vi "subAddControl.vi"(0 "Input Symbol Stream":cdb[][](array[numeric]), 9 "Training Sequence":cdb[](array[numeric])=[0.7071067811865475+0.7071067811865475i, 0.7071067811865475+0.7071067811865475i, 0.7071067811865475+0.7071067811865475i, -0.7071067811865475-0.7071067811865475i, -0.7071067811865475-0.7071067811865475i, -0.7071067811865475-0.7071067811865475i, 0.7071067811865475+0.7071067811865475i, -0.7071067811865475-0.7071067811865475i, -0.7071067811865475-0.7071067811865475i, 0.7071067811865475+0.7071067811865475i, -0.7071067811865475-0.7071067811865475i, 0.7071067811865475+0.7071067811865475i, 0.7071067811865475+0.7071067811865475i, 0.7071067811865475+0.7071067811865475i, -0.7071067811865475-0.7071067811865475i, -0.7071067811865475-0.7071067811865475i, -0.7071067811865475-0.7071067811865475i, 0.7071067811865475+0.7071067811865475i, -0.7071067811865475-0.7071067811865475i, -0.7071067811865475-0.7071067811865475i, 0.7071067811865475+0.7071067811865475i, -0.7071067811865475-0.7071067811865475i, 0.7071067811865475+0.7071067811865475i, 0.7071067811865475+0.7071067811865475i, 0.7071067811865475+0.7071067811865475i, -0.7071067811865475-0.7071067811865475i, -0.7071067811865475-0.7071067811865475i, -0.7071067811865475-0.7071067811865475i, 0.7071067811865475+0.7071067811865475i, -0.7071067811865475-0.7071067811865475i, -0.7071067811865475-0.7071067811865475i, 0.7071067811865475+0.7071067811865475i, -0.7071067811865475-0.7071067811865475i, 0.7071067811865475+0.7071067811865475i, 0.7071067811865475+0.7071067811865475i, 0.7071067811865475+0.7071067811865475i, -0.7071067811865475-0.7071067811865475i, -0.7071067811865475-0.7071067811865475i, -0.7071067811865475-0.7071067811865475i, 0.7071067811865475+0.7071067811865475i, -0.7071067811865475-0.7071067811865475i, -0.7071067811865475-0.7071067811865475i, 0.7071067811865475+0.7071067811865475i, -0.7071067811865475-0.7071067811865475i] format="%#_3p", 11 "error in (no error)":errorcluster) -> (4 "Output Transmit \nPackets":cdb[][](array[numeric]), 15 "error out":errorcluster)   [LabVIEW 2011]
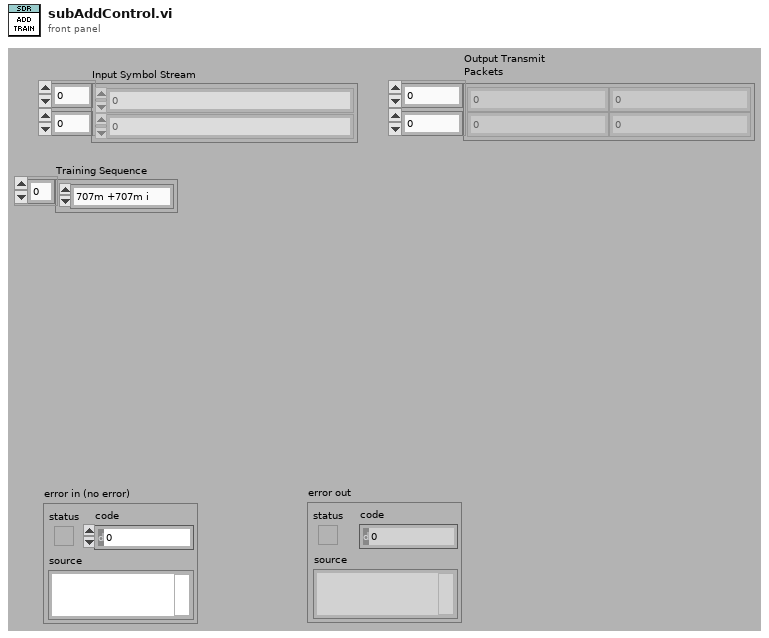
[diagram p1: front panel]
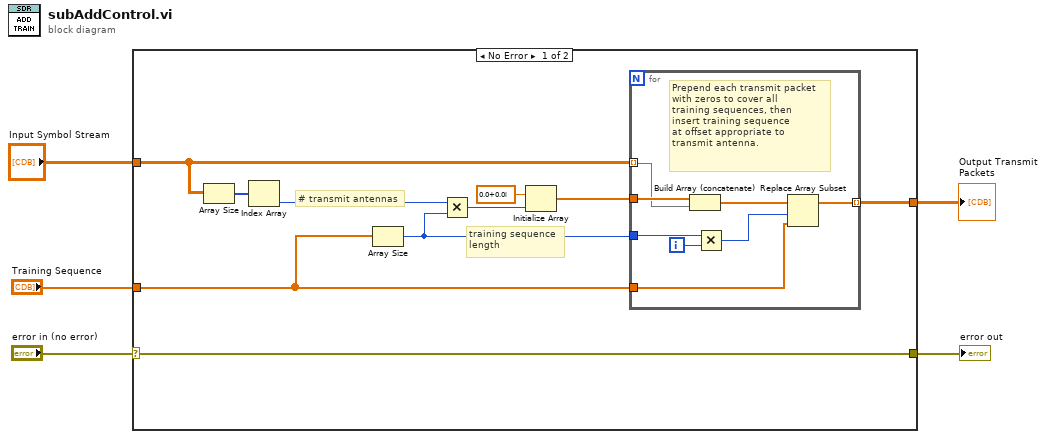
[diagram p0: block diagram]
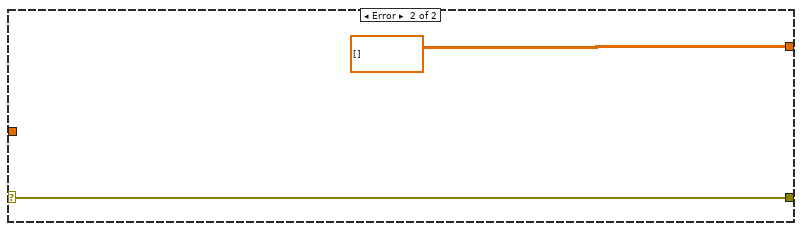
[diagram p2: hidden frame]
diagram:
  n1 = case shown="No Error" "error in (no error)" {
    selector: "error in (no error)" -> [w15 w25]
    tunnel: [w15 w25] -> w4
    tunnel: "Input Symbol Stream" -> [w13 _]
    tunnel: "Training Sequence" -> [w6 _]
    tunnel: [w7 cdb[][] []] -> w2
    frame No Error {
      # "training sequence\nlength"
      # "# transmit antennas"
      n2 = Array Size(array=w13) -> (size(s)=w12:i32[])
      n3 = Index Array(array=w12) -> (element=w11:i32)  [unwired: 1 in]
      n4 = Array Size(array=w6) -> (size(s)=w8:i32)
      n5 = Multiply(x=w11, y=w8) -> (x*y=w10:i32)
      n6 = Initialize Array(cdb 0.0+0.0i, w10) -> (w9:cdb[])
      n7 = for {
        tunnel: w13 -> [w22] mode=indexing
        tunnel: w9 -> [w23]
        tunnel: w8 -> [w20]
        tunnel: w6 -> [w18]
        tunnel: [w16] -> w7 mode=indexing
        i -> [w19]
        # "Prepend each transmit packet\nwith zeros to cover all\ntraining sequences, then \ninsert training sequence\nat offset appropriate to \ntransmit antenna."
        n8 = Build Array (concatenate)(w23, w22) -> (w21:cdb[])
        n9 = Multiply(x=w20, y=w19) -> (x*y=w17:i32)
        n10 = Replace Array Subset(array=w21, new element=w18, index=w17) -> (w16:cdb[])
      }
    }
    frame Error {
    }
  }
  "error out" <- w4
  "Output Transmit \nPackets" <- w2
